vi "Add Data.vi"(8 "Error In":errorcluster, 10 "Data":string, 11 "Message In":string) -> (0 "Error Out":errorcluster, 3 "Message Out":string)   [LabVIEW 2014, in "i3-sse-server.lvlib"]
uses:
  i3-sse-server.lvlib
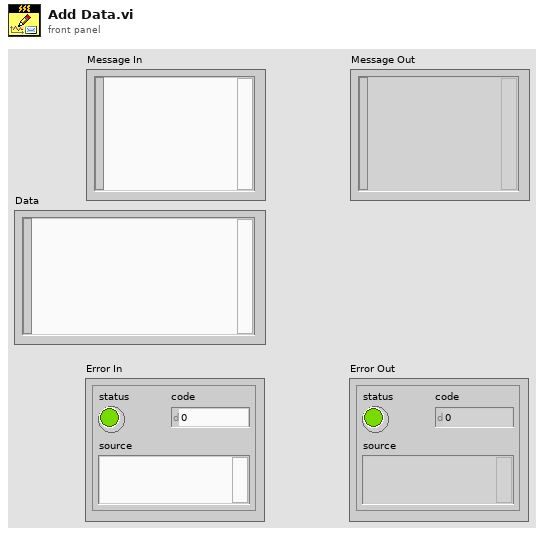
[diagram p1: front panel]
types:
  T1 = enum16{"Native", "Native Command Line", "UNIX", "Macintosh", "DOS"}
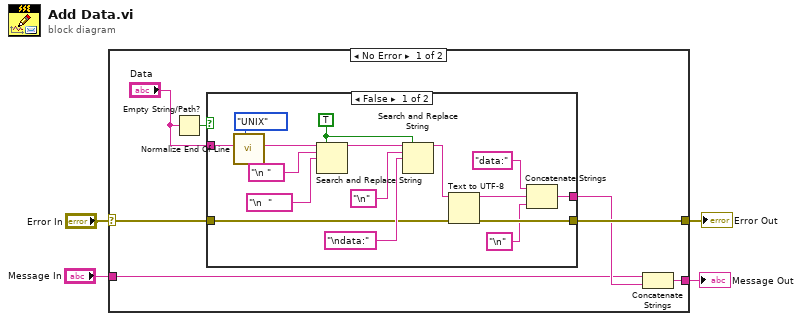
[diagram p0: block diagram]
diagram:
  n1 = case shown="No Error" "Error In" {
    selector: "Error In" -> [w9 w31]
    tunnel: [w8 w31] -> w2
    tunnel: [w7 w30] -> w3
    tunnel: "Message In" -> [w5 w30]
    frame No Error {
      n2 = Empty String/Path?(string/path="Data") -> (empty?=w11:bool)
      n3 = case shown="False" w11 {
        tunnel: "Data" -> [w27 w28]
        tunnel: w9 -> [w18 w29]
        tunnel: [w17 w29] -> w8
        tunnel: [w15 w28] -> w6
        frame False {
          w21 = TRUE ("replace all? (F)")
          n4 = call <vilib>:"Normalize End Of Line.vi"("end of line (Native)"=T1."UNIX", "string in"=w27) -> ("string out"=w25:string)  [unwired: 6 in]
          n5 = Search and Replace String(replace all?=w21, input string=w25, search string="\n ", replace string="\n  " ("replace string (\"\")")) -> (result string=w22:string)  [unwired: 4 in, 3 out]
          n6 = Search and Replace String(replace all?=w21, input string=w22, search string="\n", replace string="\ndata:" ("search string")) -> (result string=w16:string)  [unwired: 4 in, 3 out]
          n7 = Text to UTF-8(8:w18, 11:w16) -> (0:w17:errorcluster, 3:w13:string)  [unwired: 1 in]
          n8 = Concatenate Strings("data:" ("string"), w13, "\n" ("string")) -> (w15:string)
        }
        frame True {
        }
      }
      n9 = Concatenate Strings(w5, w6) -> (w7:string)
    }
    frame Error {
    }
  }
  "Error Out" <- w2
  "Message Out" <- w3
